vi "Generate Report.vi"(8 "error in (no error)":errorcluster, 10 "Resource In":variant, 11 "HIJ Vision Display in":refnum<class "HIJ Vision Display.lvclass">) -> (0 "error out":errorcluster, 2 "Resource Out":variant, 3 "HIJ Vision Display out":refnum<class "HIJ Vision Display.lvclass">)   [LabVIEW 2020, in "HIJ Vision Display.lvlib" / "HIJ Vision Display.lvclass"]
uses:
  HIJ Vision Display.lvclass
  HIJ Vision Display.lvclass/HIJ Vision Display.ctl
  Analyze/Results and Overlays/Results Base/Analyze Results Base.lvclass
  Analyze/Analyze Parameter/Analyze Parameter Base/Analyze Parameter Base.lvclass
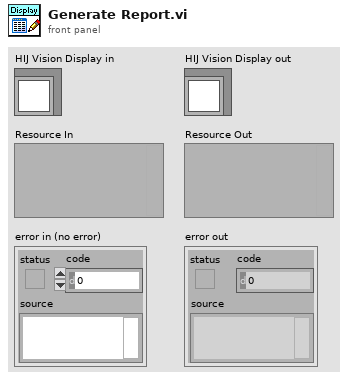
[diagram p1: front panel]
types:
  T1 = typedef "HIJ Vision Display.lvlib/HIJ Vision Display.lvclass/DisplaySettings.ctl" = cluster{"Min. Thresh.":sgl, "X":dbl, "Y":dbl, "ShowLineout":bool, "ScaleParts":i32, "ShowLegende":bool, "Target Cross":bool, "Centroid Cross":bool, "Target color":u32, "Centroid color":u32, "calibr. µm/px":sgl[unit]}
  T2 = typedef "NI_LVConfig.lvlib/Config Data RefNum.ctl" = refnum<k1>
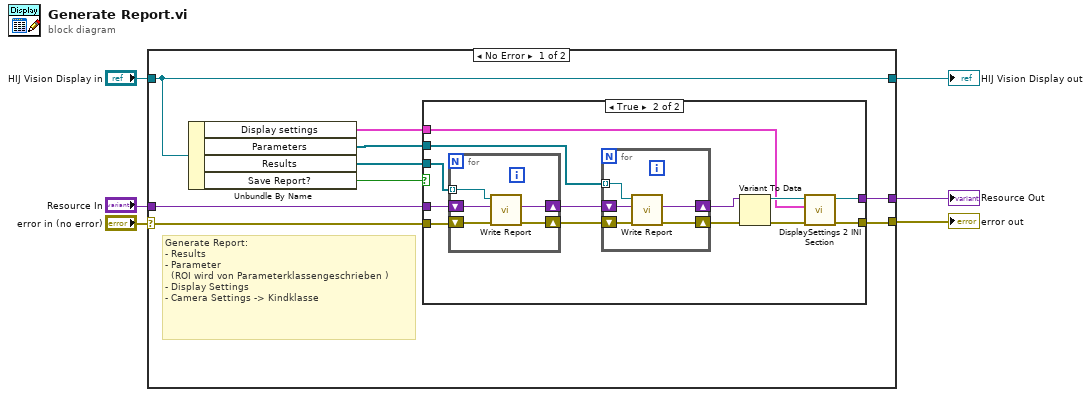
[diagram p0: block diagram]
diagram:
  n1 = case shown="No Error" "error in (no error)" {
    selector: "error in (no error)" -> [w9 w43]
    tunnel: [w10 w43] -> w5
    tunnel: [w14 w42] -> w3
    tunnel: "HIJ Vision Display in" -> [w14 w42]
    tunnel: "Resource In" -> [w15 w41]
    tunnel: [w8 w41] -> w1
    frame No Error {
      # "Generate Report:\n- Results\n- Parameter \n  (ROI wird von Parameterklassengeschrieben )\n- Display Settings\n- Camera Settings -> Kindklasse"
      n2 = Unbundle By Name(w14) -> ("Display settings"=w7:T1, "Parameters"=w11:refnum<class "Analyze Parameter Base.lvclass">[], "Results"=w12:refnum<class "Analyze Results Base.lvclass">[], "Save Report?"=w13:bool)
      n3 = case shown="True" w13 {
        tunnel: [w17 w20] -> w10
        tunnel: w12 -> [_ w30]
        tunnel: w11 -> [_ w27]
        tunnel: w9 -> [w17 w26]
        tunnel: w15 -> [w16 w25]
        tunnel: [w16 w19] -> w8
        tunnel: w7 -> [_ w18]
        frame False {
        }
        frame True {
          n4 = for {
            shift-right: [w34] -> w29
            shift-left: w26 -> [w35]
            tunnel: w30 -> [w33] mode=indexing
            shift-right: [w32] -> w28
            shift-left: w25 -> [w31]
            n5 = call-dynamic "Write Report.vi"("error in (no error)"=w35, "Resource In"=w31, "Analyze Results Base in"=w33) -> ("error out"=w34:errorcluster, "Resource Out"=w32:variant)  [unwired: 6 in, 1 out]
          }
          n6 = for {
            tunnel: w27 -> [w38] mode=indexing
            shift-right: [w37] -> w23
            shift-left: w29 -> [w40]
            shift-right: [w36] -> w24
            shift-left: w28 -> [w39]
            n7 = call-dynamic "Write Report.vi"("error in (no error)"=w40, "Resource In"=w39, "Analyze Parameter Base in"=w38) -> ("error out"=w37:errorcluster, "Resource Out"=w36:variant)  [unwired: 6 in, 1 out]
          }
          n8 = Variant To Data(error in=w23, Variant=w24) -> (data=w21:T2, error out=w22:errorcluster)  [unwired: 1 in]
          n9 = call "DisplaySettings 2 INI Section.vi"("error in (no error)"=w22, "Display settings"=w18, "refnum in"=w21) -> ("error out"=w20:errorcluster, "refnum out"=w19:T2)  [unwired: 7 in]
        }
      }
    }
    frame Error {
    }
  }
  "error out" <- w5
  "HIJ Vision Display out" <- w3
  "Resource Out" <- w1
